vi "TDMS_Open.vi"(7 "Offset":bool, 10 "Input 2D":dbl[][](array[numeric]), 11 "Open":bool) -> (1 "Output 2D":dbl[][](array[numeric]), 3 "Freq_Sampling_SizeX_SizeY":dbl[](array[numeric]))   [LabVIEW 2018]
uses:
  <vilib>/Platform/NI_3dgraph.lvlib
panel:
  out "Numeric":i32
  in  "milliseconds to wait":u32
  in  "3D Surface":refnum<k7>(container)
  in  "Samples per Channel":i32=1000 caption="Samples"
  in  "Rate":dbl=60000.0 caption="Sample Rate (Hz)" format="%0.0f"
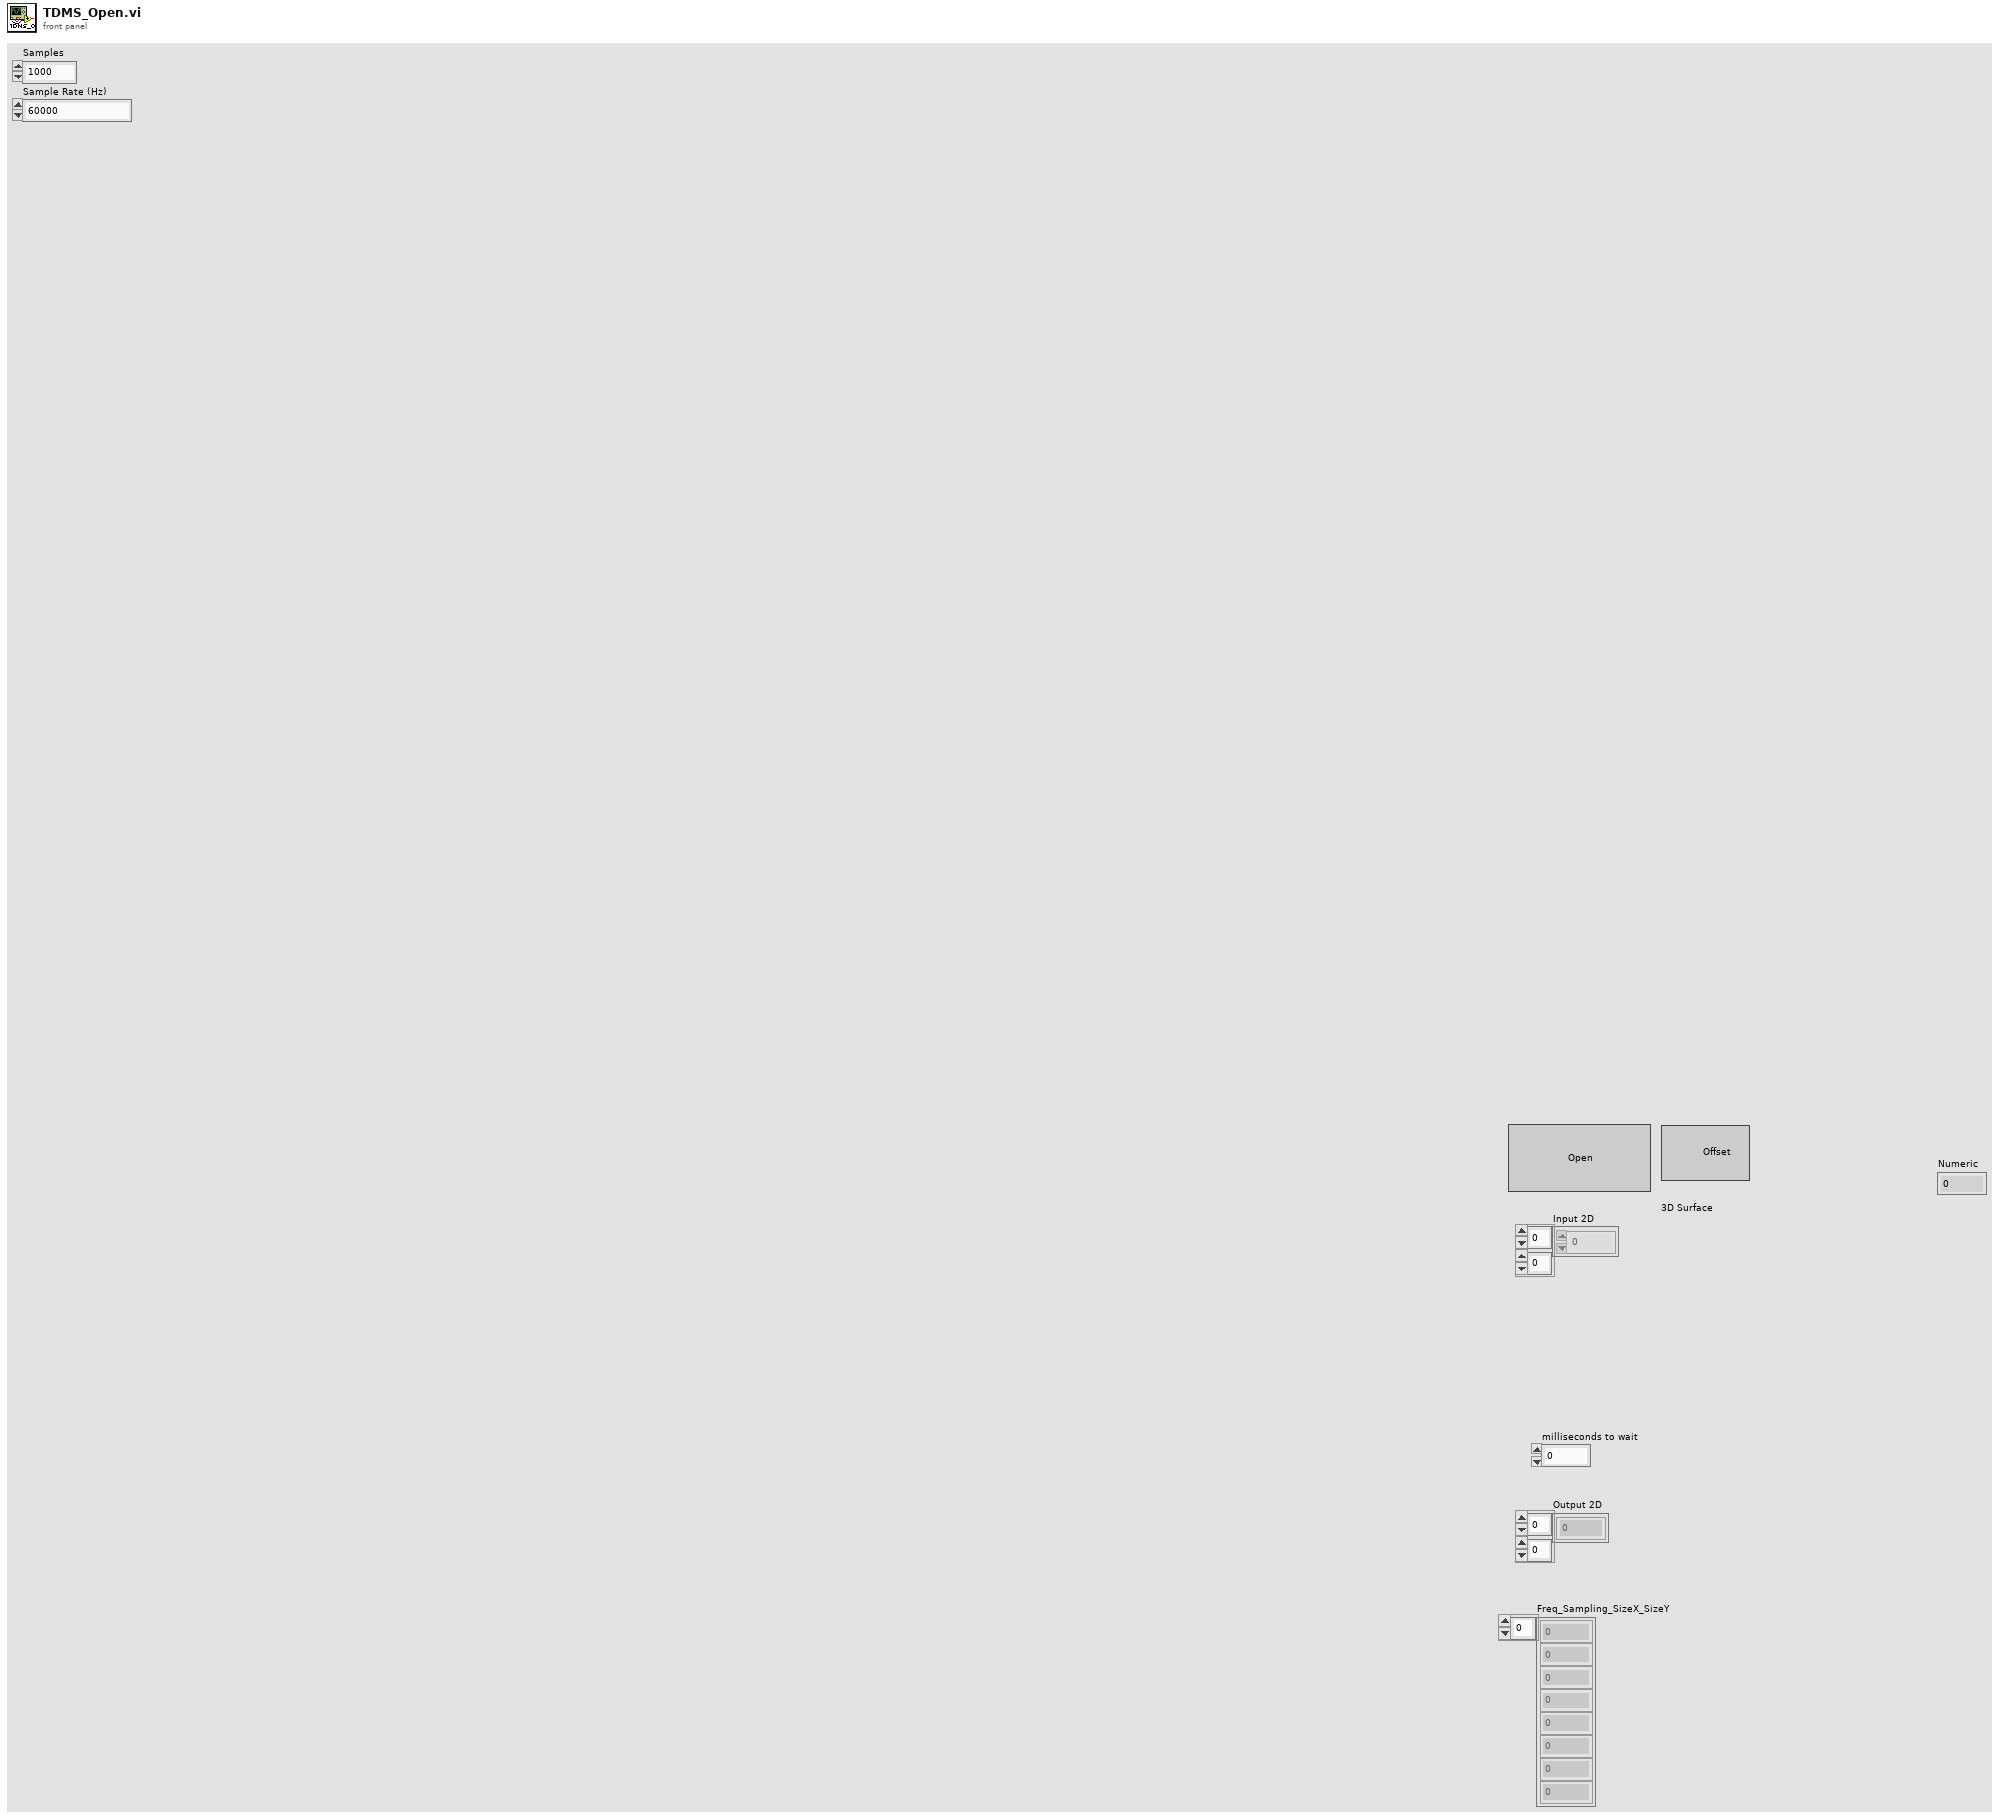
[diagram p1: front panel]
types:
  T1 = enum16{"open", "open or create", "create or replace", "create", "open (read-only)"}
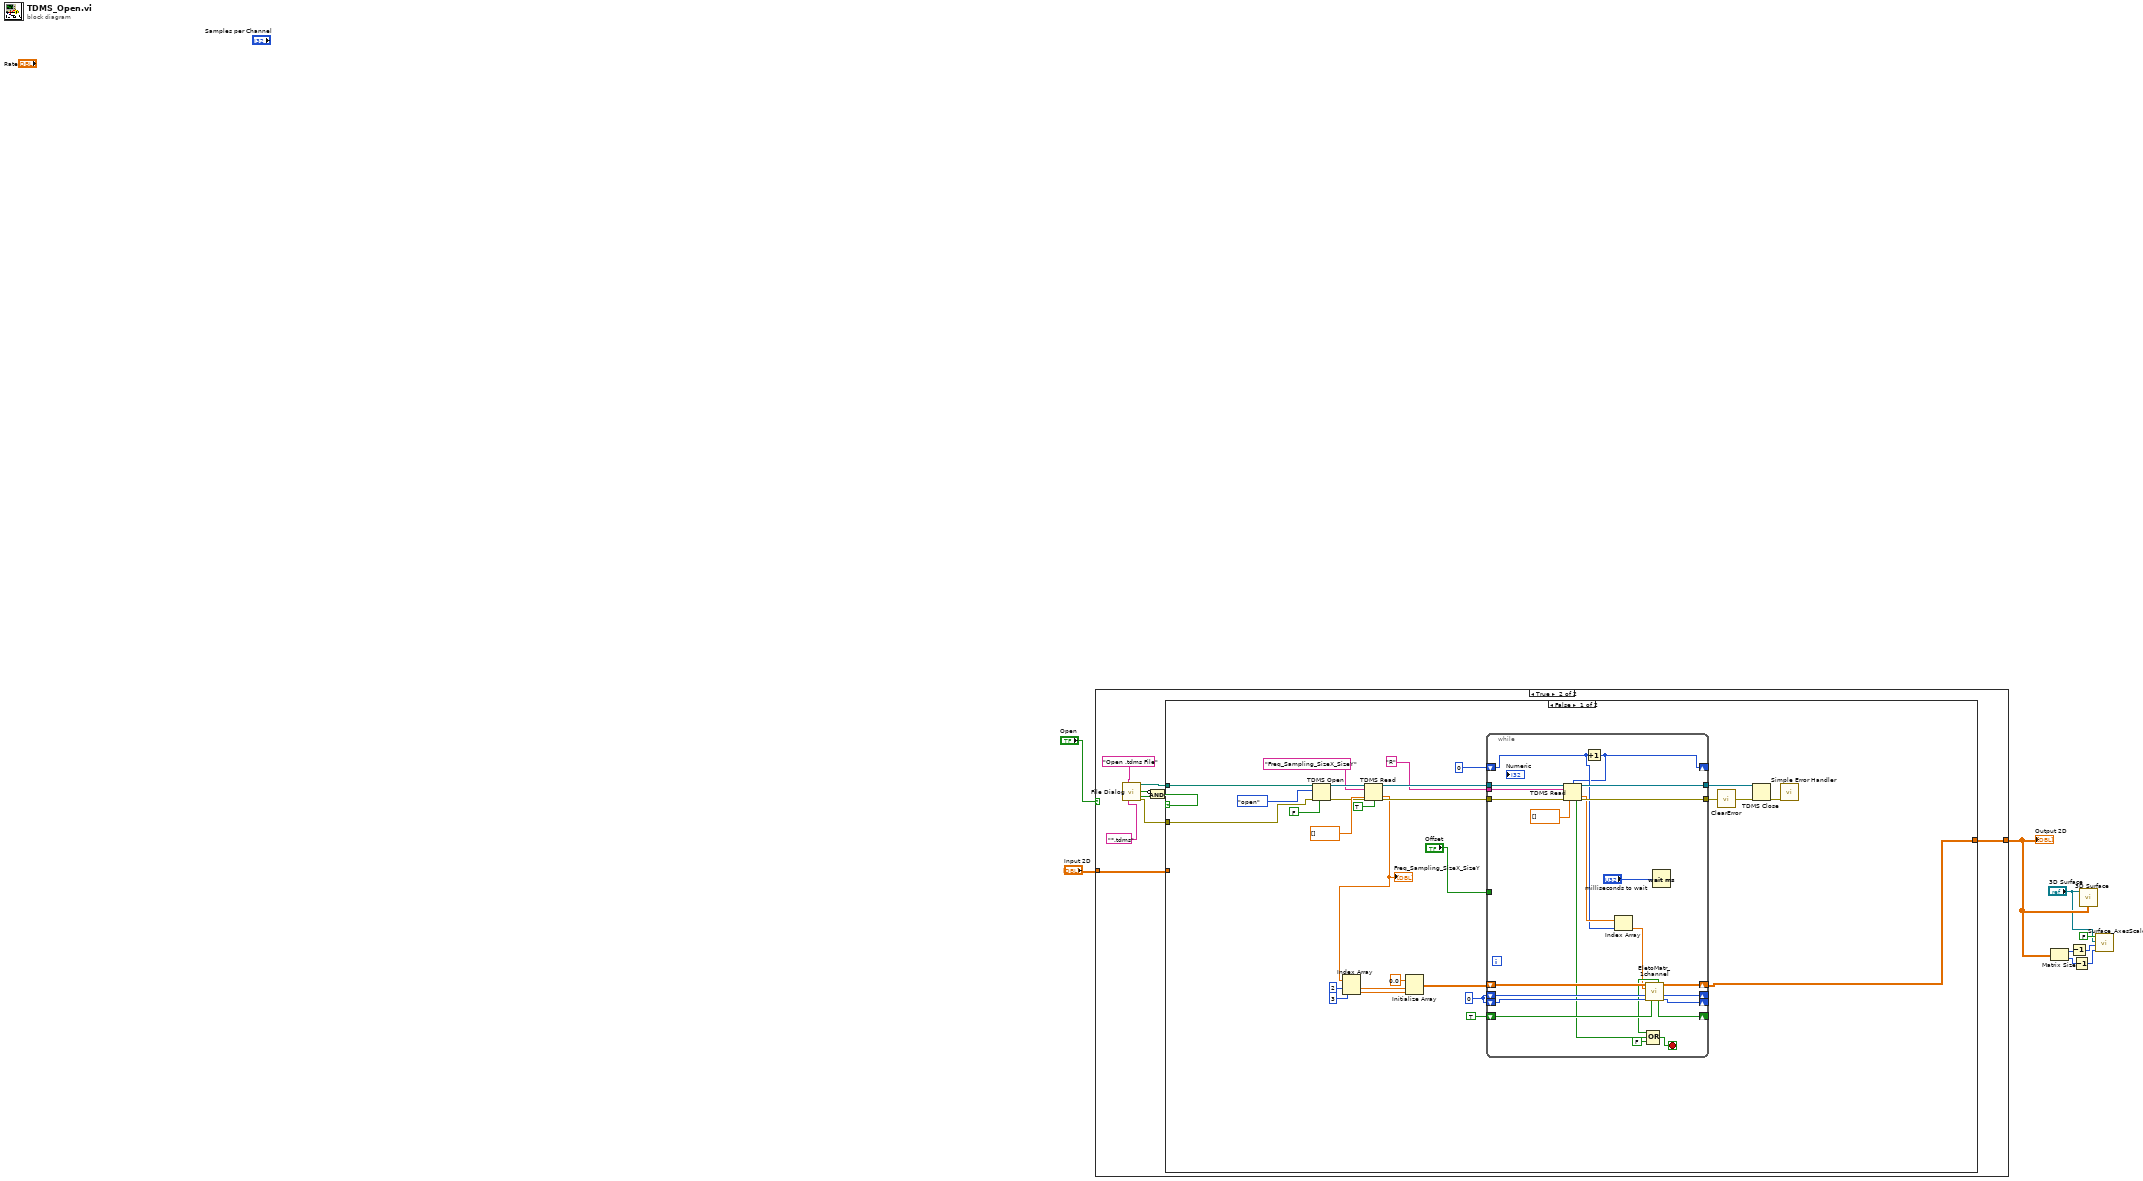
[diagram p0: block diagram]
diagram:
  n1 = case shown="True" "Open" {
    tunnel: [w10 w13] -> w4
    tunnel: "Input 2D" -> [w10 w12]
    frame False {
    }
    frame True {
      n2 = call "File Dialog"("prompt"="Open .tdms File" ("button label"), "pattern (all files)"="*.tdms") -> ("selected path"=w19:path, "exists"=w17:bool, "cancelled"=w16:bool, "error out"=w11:errorcluster)  [unwired: 10 in]
      n3 = Compound Arithmetic op=AND(invert w17, w16) -> (w15:bool)
      n4 = case shown="False" w15 {
        tunnel: w19 -> [w23 _]
        tunnel: [w22 w71] -> w13
        tunnel: w12 -> [_ w71]
        tunnel: w11 -> [w37 _]
        frame False {
          w29 = 0 ("Out Row")
          n5 = TDMS Open(6:FALSE ("disable buffering (T)"), 8:w37, 10:T1."open" ("operation"), 11:w23) -> (0:w43:errorcluster, 3:w47:refnum<k34>)  [unwired: 3 in]
          n6 = TDMS Read(0:w47, 5:"Freq_Sampling_SizeX_SizeY" ("group name in"), 11:w43, 12:dbl[] [] ("Array"), 13:TRUE ("return channels in file order? (F)")) -> (4:w27:refnum<k34>, 10:w21:dbl[], 15:w36:errorcluster)  [unwired: 3 in, 3 out]
          "Freq_Sampling_SizeX_SizeY" <- w21
          n7 = Index Array(array=w21, index #1=2 ("index"), index #2=3 ("index")) -> (element #1=w31:dbl, element #2=w30:dbl)
          n8 = Initialize Array(0.0 ("element"), w31, w30) -> (w32:dbl[][])
          n9 = while {
            tunnel: [w70] -> w39
            tunnel: [w69] -> w38
            tunnel: "R" ("group name in") -> [w56]
            tunnel: w27 -> [w67]
            tunnel: w36 -> [w66]
            shift-right: [w64] -> w22
            shift-left: w32 -> [w65]
            shift-right: [w61] -> _
            shift-left: w29 -> [w63]
            shift-right: [w60] -> _
            shift-left: w29 -> [w62]
            shift-right: [w58] -> _
            shift-left: TRUE ("Output Direction") -> [w59]
            tunnel: "Offset" -> [_]
            shift-right: [w48] -> _
            shift-left: 0 -> [w49]
            stop <- w53 stop-if-true
            n10 = Increment(x=w49) -> (x+1=w48:i32)
            n11 = TDMS Read(0:w67, 2:w48, 5:w56, 11:w66, 12:dbl[] [] ("Array")) -> (4:w70:refnum<k34>, 10:w51:dbl[], 14:w54:bool, 15:w69:errorcluster)  [unwired: 3 in, 2 out]
            n12 = Index Array(array=w51, index=w49) -> (element=w50:dbl)
            n13 = call "EletoMatr_1channel.vi"("Input Array X"=w65, "Input data"=w50, "In Row"=w63, "In Column"=w62, "Input Direction"=w59) -> ("Completed"=w55:bool, "Out Array X"=w64:dbl[][], "Out Row"=w61:i32, "Output Direction"=w58:bool, "Out Column"=w60:i32)  [unwired: 6 in]
            n14 = Compound Arithmetic op=OR(w55, w54, FALSE ("value")) -> (w53:bool)
            n15 = Wait (ms)(milliseconds to wait="milliseconds to wait") -> ()  [unwired: 1 out]
          }
          n16 = call <vilib>:"ClearError.vi"("error in (no error)"=w38) -> ("error out"=w41:errorcluster)
          n17 = TDMS Close(8:w41, 11:w39) -> (0:w40:errorcluster)  [unwired: 1 out]
          n18 = call <vilib>:"Simple Error Handler.vi"("error in (no error)"=w40) -> ()  [unwired: 1 in, 8 out]
        }
        frame True {
        }
      }
    }
  }
  "Output 2D" <- w4
  n19 = Matrix Size(0:w4) -> (1:w5:i32, 2:w2:i32)
  n20 = Decrement(x=w5) -> (x-1=w7:i32)
  n21 = Decrement(x=w2) -> (x-1=w1:i32)
  n22 = call <vilib>:"3D Surface.vi"("z matrix"=w4, "3D graph"="3D Surface") -> ()  [unwired: 8 in, 2 out]
  n23 = call "Surface_AxesScale.vi"("Y-axis Max"=w1, "X-axis max"=w7, "3D Surface"="3D Surface", "Auto Scale"=FALSE) -> ()  [unwired: 8 in]
